vi "Mandelbrot_Top.vi"() -> ()   [LabVIEW 2020]
doc: "This benchmark is designed to demonstrate execution performance improvement when executing FFT and IFFT operations on a GPU."
uses:
  <vilib>/Analysis/baseanly.llb/Mean (DBL).vi
  <vilib>/Analysis/1siggen.llb/Ramp Pattern by Delta.vi
  <vilib>/Utility/file.llb/Read Delimited Spreadsheet (DBL).vi
  <vilib>/Ngene/CuLab - GPU Accelerated Toolkit/Toolkit/CuLab.lvlib
  <vilib>/Analysis/NI_AALBase.lvlib
panel:
  out "CuLab Mean Performance Gain":dbl[](array[numeric])=[1.0, 22.05888198839261, 2.294988144455706] format="%#.2g"
  out "Releative Exec Time vs CuLab (smaller is better)":cluster{i32[], "all rows":dbl[]}[](graph)=[{[100, 200, 300, 400, 500, 600, 700, 800, 900, 1000], "all rows"=[1.0, 1.0, 1.0, 1.0, 1.0, 1.0, 1.0, 1.0, 1.0, 1.0]}, {[100, 200, 300, 400, 500, 600, 700, 800, 900, 1000], "all rows"=[0.8045912431423006, 2.8737294623342633, 6.2281949138049875, 11.291126277991692, 18.815012396949246, 27.10316550048527, 34.90172708957351, 38.99811295548449, 39.49387679077455, 40.07928325338579]}, {[100, 200, 300, 400, 500, 600, 700, 800, 900, 1000], "all rows"=[2.9876362098895357, 2.6173252742418085, 2.4274383662643, 2.414197215437082, 2.5477456703897334, 2.477240832223878, 2.3481639475839504, 2.0064648536535485, 1.786744893645114, 1.336924181228108]}]
  in  "CuPy CSV":path=path "D:/Ngene/GitHub/culab_examples/Benchmarks/CuPy/results/GeForce_RTX_2080_Ti/Mandelbrot_CuPy.csv"
  out "Execution Time":cluster{i32[], "FFT mean Exec Time":dbl[]}[](graph)=[{[100, 200, 300, 400, 500, 600, 700, 800, 900, 1000], "FFT mean Exec Time"=[0.1258352000004379, 0.13859289999982138, 0.1453709000006711, 0.14599060000000463, 0.1388639000006151, 0.14194279999992432, 0.1489036999992095, 0.17667840000012802, 0.22171379999963392, 0.26985270000022865]}, {[100, 200, 300, 400, 500, 600, 700, 800, 900, 1000], "FFT mean Exec Time"=[0.10124589999941236, 0.398278499999833, 0.9053982999994332, 1.6483982999998261, 2.6127260000002934, 3.8470992000002298, 5.196996300000137, 6.8901241999992635, 8.756337499999972, 10.815502800000104]}, {[100, 200, 300, 400, 500, 600, 700, 800, 900, 1000], "FFT mean Exec Time"=[0.3759498, 0.36274270000000003, 0.3528789, 0.35245010000000004, 0.35378990000000005, 0.3516265, 0.3496503, 0.354499, 0.396146, 0.3607726]}]
  in  "Size Delta":i32=100
  out "GPU Model":string="NVIDIA GeForce RTX 2080 Ti"
  out "CPU Model":string="Intel(R) Core(TM) i7-8700K"
  in  "Max Iterations":i32=1000
  in  "Size Stop":i32=1000
  in  "Size Start":i32=100
  out "Dims H,W":i32[](array[numeric])=[100, 200, 300, 400, 500, 600, 700, 800, 900, 1000] format="%.2p"
  # "Mandelbrot Benchmark"
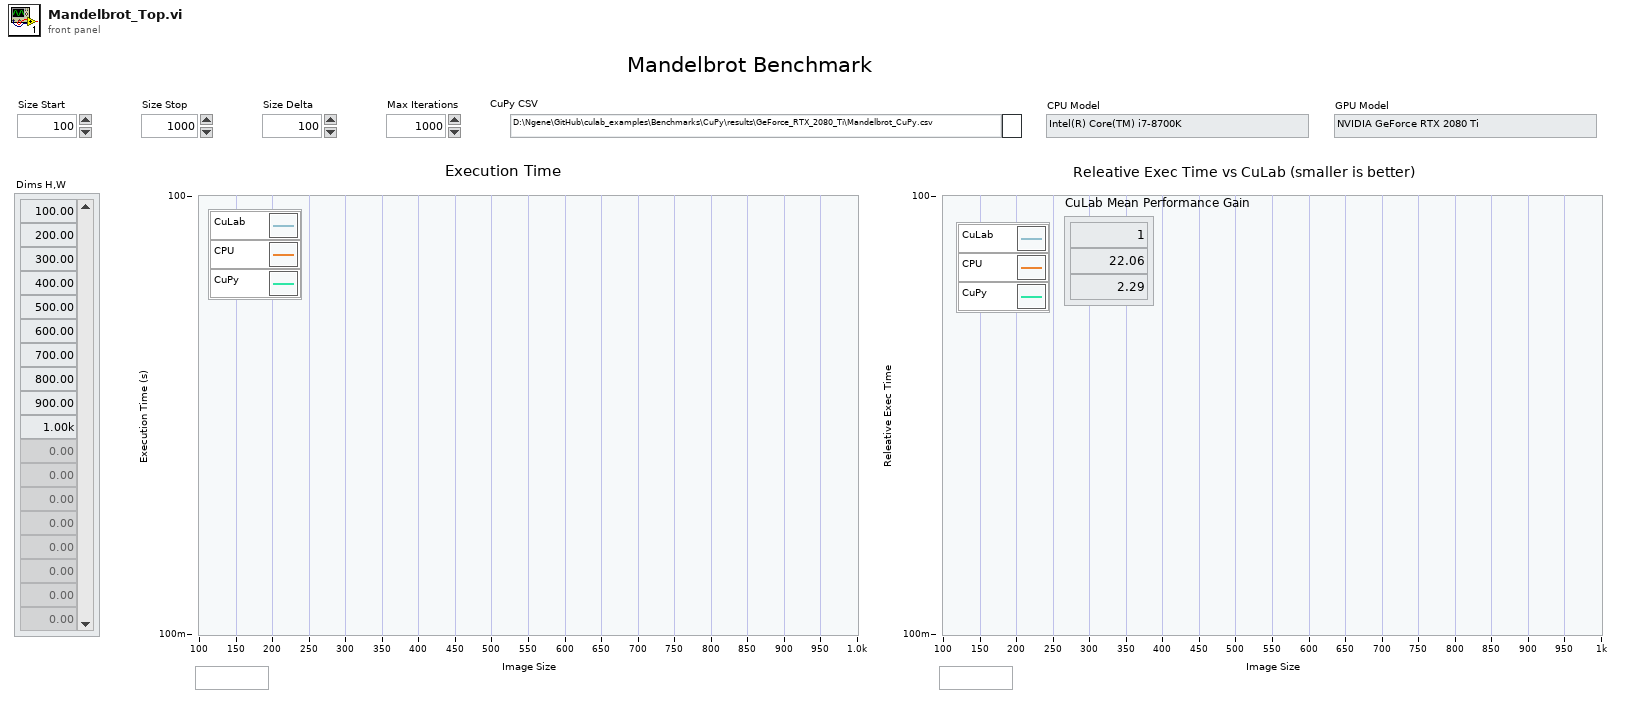
[diagram p1: front panel]
types:
  T1 = typedef "CuLab.lvlib/Properties.ctl" = cluster{"Device ID":i32, "Name":string}
  T2 = typedef "imagedata.ctl" = cluster{"image type":i32, "image depth":i32, "image":u8[], "mask":u8[], "colors":u32[], "Rectangle":cluster{"left":i16, "top":i16, "right":i16, "bottom":i16}}
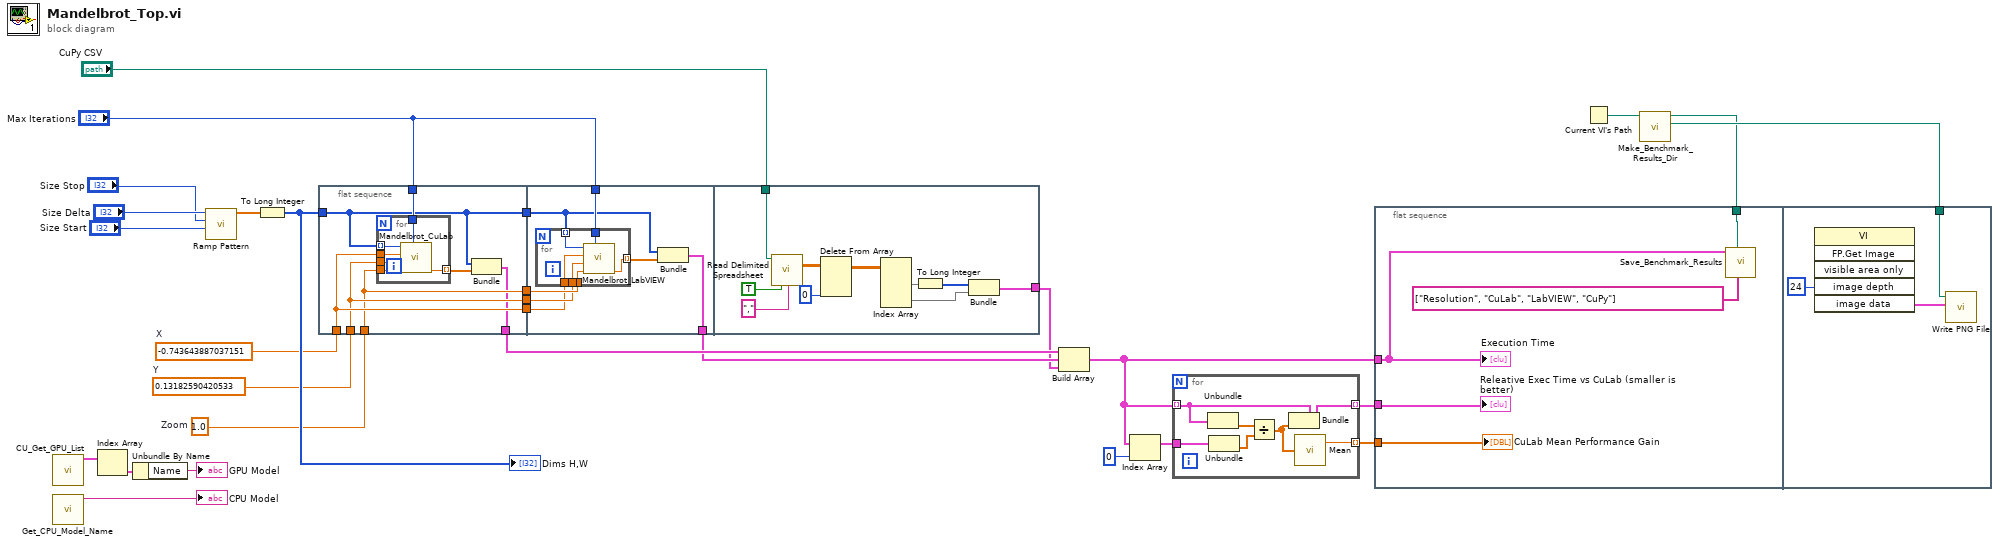
[diagram p0: block diagram]
diagram:
  w17 = 1.0  # Zoom
  w18 = 0.13182590420533  # Y
  w19 = -0.743643887037151  # X
  n1 = call <vilib>:"CU_Get_GPU_List.vi"() -> ("Devices"=w28:T1[])  [unwired: 10 in, 1 out]
  n2 = call "Get_CPU_Model_Name.vi"() -> ("CPU Model"=→"CPU Model":string)  [unwired: 11 in]
  n3 = Index Array(array=w28) -> (element=w27:T1)  [unwired: 1 in]
  n4 = Unbundle By Name(w27) -> ("Name"=→"GPU Model":string)
  n5 = call-poly <vilib>:"Ramp Pattern.vi"("start"="Size Start", "end"="Size Stop", "delta"="Size Delta") -> ("Ramp Pattern"=w21:dbl[])  [unwired: 6 in, 2 out]
  n6 = To Long Integer(number=w21) -> (32bit integer=w20:i32[])
  "Dims H,W" <- w20
  n7 = flat-sequence {
    tunnel: [w30] -> w25
    tunnel: [w31] -> w26
    tunnel: w20 -> [w31]
    tunnel: "Max Iterations" -> [w36]
    tunnel: w19 -> [w35]
    tunnel: w18 -> [w34]
    tunnel: w17 -> [w33]
    tunnel: [w35] -> w16
    tunnel: [w34] -> w15
    tunnel: [w33] -> w14
    tunnel: w26 -> [w44]
    tunnel: "Max Iterations" -> [w49]
    tunnel: w16 -> [w46]
    tunnel: w15 -> [w47]
    tunnel: w14 -> [w48]
    tunnel: [w43] -> w12
    tunnel: "CuPy CSV" -> [w65]
    tunnel: [w57] -> w8
    frame #0 {
      n8 = for {
        tunnel: w36 -> [w42]
        tunnel: w35 -> [w41]
        tunnel: w34 -> [w40]
        tunnel: w33 -> [w39]
        tunnel: w31 -> [w37] mode=indexing
        tunnel: [w38] -> w32 mode=indexing
        n9 = call "Mandelbrot_CuLab.vi"("Max_iter"=w42, "Zoom"=w39, "y"=w40, "x"=w41, "Resolution"=w37) -> ("Exec Time"=w38:dbl)  [unwired: 5 in, 1 out]
      }
      n10 = Bundle(w31, w32) -> (w30:cluster{i32[], dbl[]})  [unwired: 1 in]
    }
    frame #1 {
      n11 = for {
        tunnel: w44 -> [w55] mode=indexing
        tunnel: w49 -> [w54]
        tunnel: w48 -> [w53]
        tunnel: w47 -> [w52]
        tunnel: w46 -> [w51]
        tunnel: [w50] -> w45 mode=indexing
        n12 = call "Mandelbrot_LabVIEW.vi"("Max_iter"=w54, "Zoom"=w53, "y"=w52, "x"=w51, "Resolution"=w55) -> ("Exec Time"=w50:dbl)  [unwired: 5 in, 1 out]
      }
      n13 = Bundle(w44, w45) -> (w43:cluster{i32[], dbl[]})  [unwired: 1 in]
    }
    frame #2 {
      n14 = call-poly <vilib>:"Read Delimited Spreadsheet.vi"("file path (dialog if empty)"=w65, "transpose? (F)"=TRUE, "delimiter (\\t)"="," ("delimiter (\\t)")) -> ("all rows"=w63:dbl[][])  [unwired: 7 in, 5 out]
      n15 = Delete From Array(array=w63, index (col)=0 ("disabled index (col)")) -> (array with subset deleted=w61:dbl[][])  [unwired: 2 in, 1 out]
      n16 = Index Array(array=w61) -> (element #1=w60:dbl[], element #2=w58:dbl[])  [unwired: 4 in]
      n17 = To Long Integer(number=w60) -> (32bit integer=w59:i32[])
      n18 = Bundle(w59, "all rows"=w58) -> (w57:cluster{i32[], "all rows":dbl[]})  [unwired: 1 in]
    }
  }
  n19 = Build Array(w25, w12, w8) -> (w3:cluster{i32[], "all rows":dbl[]}[])
  n20 = Index Array(array=w3, index=0) -> (element=w11:cluster{i32[], "all rows":dbl[]})
  n21 = for {
    tunnel: w3 -> [w72] mode=indexing
    tunnel: w11 -> [w70]
    tunnel: [w71] -> w6 mode=indexing
    tunnel: [w66] -> w5 mode=indexing
    n22 = Unbundle(w72) -> ("all rows"=w69:dbl[])  [unwired: 1 out]
    n23 = Unbundle(w70) -> ("all rows"=w68:dbl[])  [unwired: 1 out]
    n24 = Divide(x=w69, y=w68) -> (x/y=w67:dbl[])
    n25 = Bundle(cluster=w72, "all rows"=w67) -> (w71:cluster{i32[], "all rows":dbl[]})  [unwired: 1 in]
    n26 = call-poly <vilib>:"Mean.vi"("X"=w67) -> ("mean"=w66:dbl)  [unwired: 1 out]
  }
  n27 = flat-sequence {
    tunnel: w6 -> [w77]
    tunnel: w5 -> [w76]
    tunnel: w3 -> [w73]
    tunnel: w4 -> [w74]
    tunnel: w7 -> [w79]
    frame #0 {
      n28 = call "Save_Benchmark_Results.vi"("Header"=string[] ["Resolution", "CuLab", "LabVIEW", "CuPy"], "file path (dialog if empty)"=w74, "Execution Time"=w73) -> ()  [unwired: 9 in]
      "Execution Time" <- w73
      "CuLab Mean Performance Gain" <- w76
      "Releative Exec Time vs CuLab (smaller is better)" <- w77
    }
    frame #1 {
      n29 = invoke class="VI" method="FP.Get Image"("image depth"=24 ("Image Depth")) -> ("image data"=w80:T2)  [unwired: 5 in, 5 out]
      n30 = call <vilib>:"Write PNG File.vi"("image data"=w80, "path to PNG file"=w79) -> ()  [unwired: 8 in, 2 out]
    }
  }
  n31 = Current VI's Path() -> (path=w1:path)
  n32 = call "Make_Benchmark_Results_Dir.vi"("Caller Path"=w1) -> ("Caller FP Image Path"=w7:path, "CSV_File"=w4:path)  [unwired: 9 in]
